vi "Read owner-id.vi"(11 "TestManagerMsg in":refnum<class "TestManagerMsg.lvclass">) -> (2 "owner-id":string, 3 "TestManagerMsg out":refnum<class "TestManagerMsg.lvclass">)   [LabVIEW 2013, in "Caraya.lvlib" / "TestManagerMsg.lvclass"]
uses:
  TestManagerMsg.lvclass
  TestManagerMsg.lvclass/TestManagerMsg.ctl
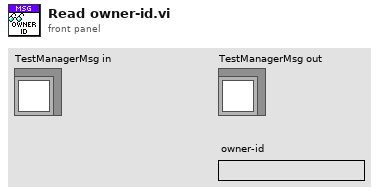
[diagram p1: front panel]
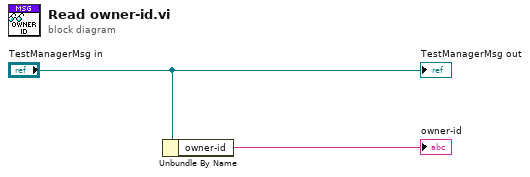
[diagram p0: block diagram]
diagram:
  n1 = Unbundle By Name("TestManagerMsg in") -> ("owner-id"=→"owner-id":string)
  "TestManagerMsg out" <- "TestManagerMsg in"
